vi "control v3.vi"() -> ()   [LabVIEW 2010]
uses:
  CaseControl.ctl
  <vilib>/Analysis/NI_AALBase.lvlib
panel:
  out "Señal de Control":dbl[](array[numeric])
  out "Arreglo de Salida":dbl[](array[numeric])
  in  "Reset":bool=TRUE
  in  "Sound Parameters":cluster{"# samples":u32, "tiempos (ms)":dbl}
  in  "Parametros Maximos":T1
  in  "detla Parametros":T1
  in  "Parametros Control":T2
  in  "Contraste":dbl
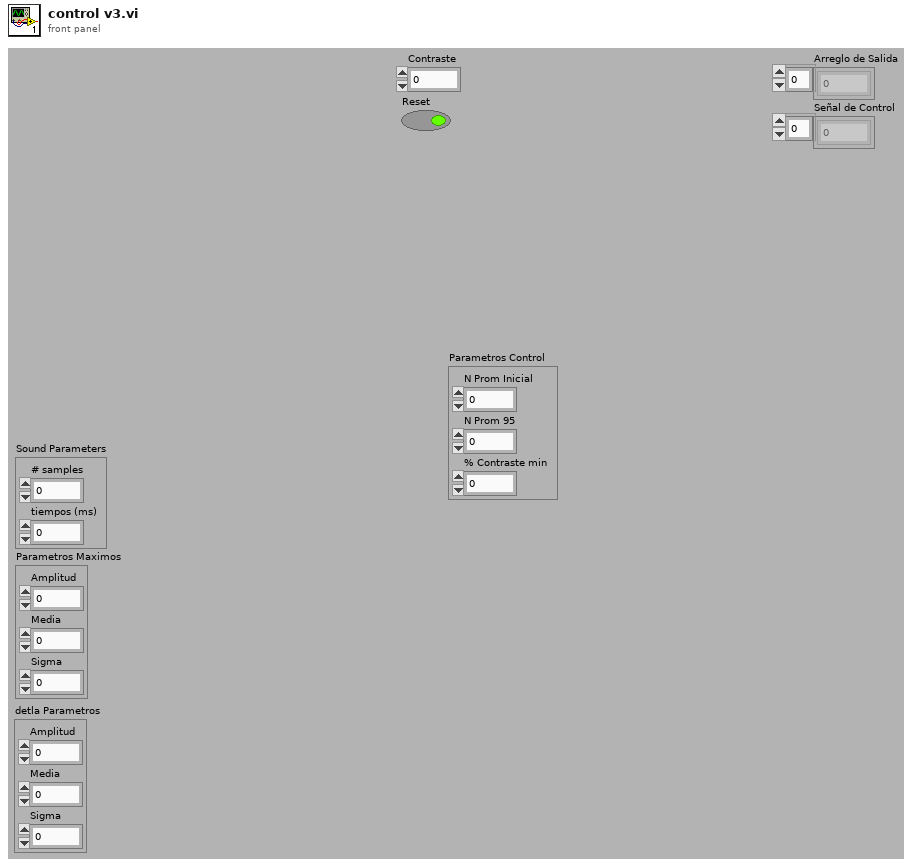
[diagram p1: front panel]
types:
  T1 = cluster{"Amplitud":dbl, "Media":dbl, "Sigma":dbl}
  T2 = cluster{"N Prom Inicial":u32, "N Prom 95":u32, "% Contraste min":dbl}
  T3 = typedef "CaseControl.ctl" = u32
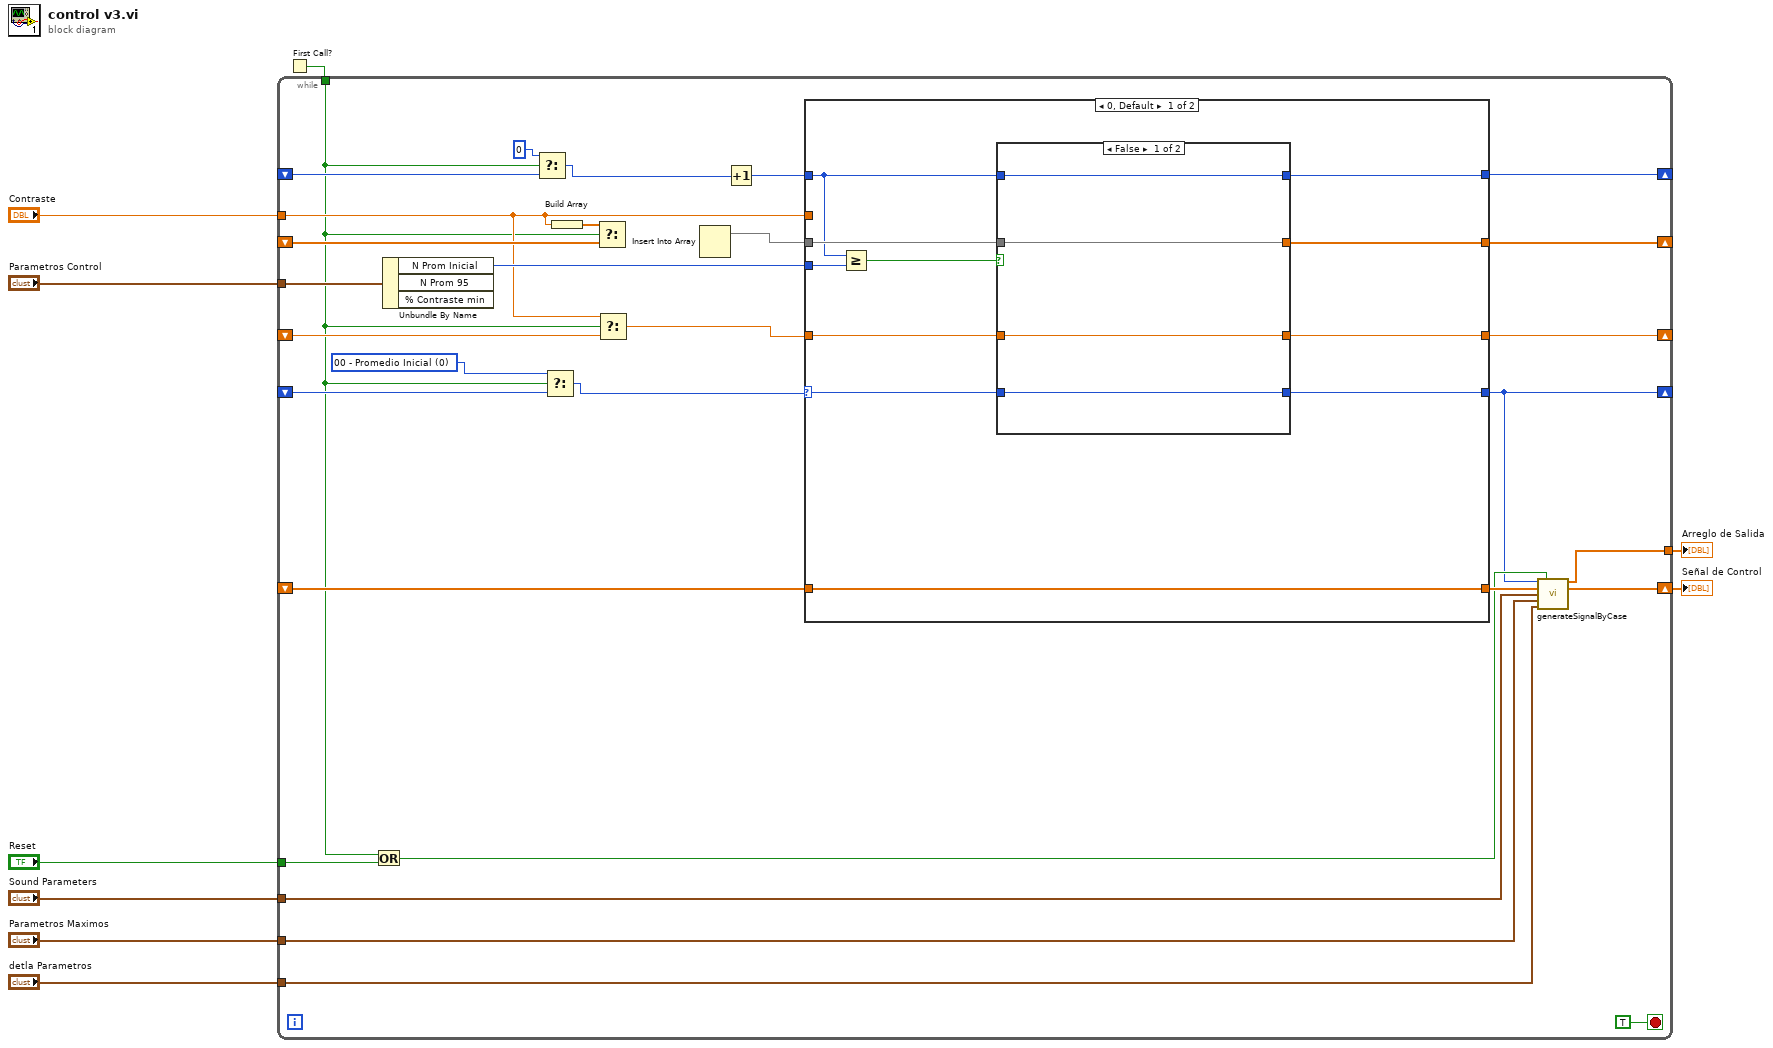
[diagram p0: block diagram]
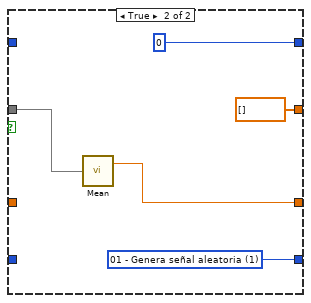
[diagram p2: hidden frame]
diagram:
  n1 = First Call?() -> (First Call?: T/F=w9:bool)
  n2 = while {
    tunnel: w9 -> [w13]
    tunnel: "Contraste" -> [w26]
    tunnel: "Parametros Control" -> [w38]
    tunnel: "Sound Parameters" -> [w18]
    tunnel: "Parametros Maximos" -> [w17]
    tunnel: "detla Parametros" -> [w16]
    shift-right: [w22] -> w1
    shift-left: _ -> [w20]
    tunnel: "Reset" -> [w37]
    shift-right: [w11] -> _
    shift-left: _ -> [w15]
    shift-right: [w34] -> _
    shift-left: _ -> [w36]
    shift-right: [w30] -> _
    shift-left: _ -> [w31]
    shift-right: [w29] -> _
    shift-left: _ -> [w28]
    tunnel: [w23] -> w2
    stop <- TRUE stop-if-true
    w12 = T3 0 items=["00 - Promedio Inicial", "01 - Genera señal aleatoria", "02 - Incrementa t0", "03 - Promedia buen t0", "04 - Inicializa Amplitud", "05 - Incrementa Amplitud", "06 - Promedia buena Amplitud", "07 - Inicializa Sigma", "08 - Incrementa Sigma", "09 - Promedia buen Sigma", "10 - Actualiza mejor señal", "11 - Control ON, Ajuste OFF", "12 - Control OFF"] ("ControlCase")
    n3 = Or(x=w13, y=w37) -> (x .or. y?=w19:bool)
    n4 = Unbundle By Name(w38) -> ("N Prom Inicial"=w33:u32)  [unwired: 2 out]
    n5 = Select(t=u32 0, s=w13, f=w36) -> (s? t:f=w25:u32)
    n6 = Select(t=w12, s=w13, f=w15) -> (s? t:f=w14:T3)
    n7 = Build Array(w26) -> (w32:dbl[])
    n8 = Select(t=w32, s=w13, f=w31) -> ()  [unwired: 1 out]
    n9 = Select(t=w26, s=w13, f=w28) -> (s? t:f=w27:dbl)
    n10 = Insert Into Array() -> (w10)  [unwired: 3 in]
    n11 = Increment(x=w25) -> (x+1=w24:u32)
    n12 = case shown="0, Default" w14 {
      selector: w14 -> [w43 _]
      tunnel: w26 -> [_ _]
      tunnel: w20 -> [w40 w61]
      tunnel: [w40 w61] -> w21
      tunnel: [w45 w60] -> w34
      tunnel: w33 -> [w50 _]
      tunnel: [w41 _] -> w11
      tunnel: w10 -> [w49 _]
      tunnel: [w42 _] -> w30
      tunnel: [w46 _] -> w29
      tunnel: w27 -> [w47 _]
      tunnel: w24 -> [w44 w60]
      frame 0, Default {
        n13 = Greater Or Equal?(x=w44, y=w50) -> (x >= y?=w48:bool)
        n14 = case shown="False" w48 {
          tunnel: w49 -> [w51 w56]
          tunnel: [w54 w59] -> w46
          tunnel: w47 -> [w54 _]
          tunnel: w44 -> [w53 _]
          tunnel: [w53 u32 0 ("t")] -> w45
          tunnel: [w52 w57] -> w41
          tunnel: w43 -> [w52 _]
          tunnel: [w51 dbl[] []] -> w42
          frame False {
          }
          frame True {
            w57 = T3 1 items=["00 - Promedio Inicial", "01 - Genera señal aleatoria", "02 - Incrementa t0", "03 - Promedia buen t0", "04 - Inicializa Amplitud", "05 - Incrementa Amplitud", "06 - Promedia buena Amplitud", "07 - Inicializa Sigma", "08 - Incrementa Sigma", "09 - Promedia buen Sigma", "10 - Actualiza mejor señal", "11 - Control ON, Ajuste OFF", "12 - Control OFF"] ("ControlCase")
            n15 = call <vilib>:"Mean.vi"("X"=w56) -> ("mean"=w59:dbl)  [unwired: 1 out]
          }
        }
      }
      frame 1 {
      }
    }
    n16 = call "generateSignalByCase.vi"("ControlCase"=w11, "Reset Control"=w19, "Señal de Control IN"=w21, "Sound Parameters"=w18, "Parametros Maximos"=w17, "detla Parametros"=w16) -> ("Arreglo de Salida"=w23:dbl[], "Señal de Control OUT"=w22:dbl[])  [unwired: 6 in, 2 out]
  }
  "Arreglo de Salida" <- w2
  "Señal de Control" <- w1
